vi "H5Pset_fapl_sec2.vi"(8 "error in (no error)":errorcluster, 11 "plist in":i32) -> (0 "error out":errorcluster, 3 "plist out":i32)   [LabVIEW 2010, in "HDF5.lvlib"]
uses:
  HDF5.lvlib
  hdf5dll.dll
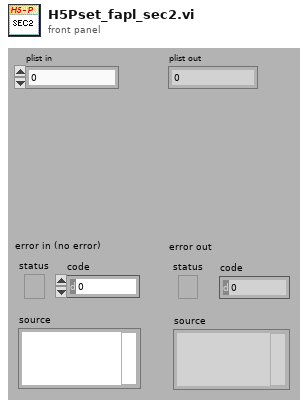
[diagram p1: front panel]
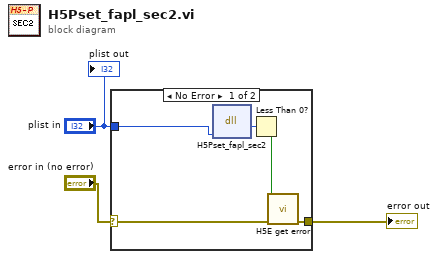
[diagram p0: block diagram]
diagram:
  n1 = case shown="No Error" "error in (no error)" {
    selector: "error in (no error)" -> [w5 w9]
    tunnel: "plist in" -> [w8 _]
    tunnel: [w4 w9] -> w2
    frame No Error {
      n2 = dll-call lib="Z:/libraries/Labview/HDF5/hdf5dll.dll" fn="H5Pset_fapl_sec2"("fapl_id"=w8) -> (w6:i32)  [unwired: 4 in, 2 out]
      n3 = Less Than 0?(x=w6) -> (x < 0?=w7:bool)
      n4 = call "H5E get error.vi"("error in (no error)"=w5, "error?"=w7) -> ("error out"=w4:errorcluster)  [unwired: 9 out]
    }
    frame Error {
    }
  }
  "error out" <- w2
  "plist out" <- "plist in"
